vi "Build Proccess JSON creation.vi"(8 "error in (no error)":errorcluster, 9 "Project Path":path, 10 "Destination Path":path, 11 "Build Specification Name":string) -> (0 "error out":errorcluster)   [LabVIEW 2023, in "Utilities.lvlib"]
uses:
  Utilities.lvlib
  <vilib>/xml/Load XML File.vi
  <vilib>/xml/NI_XML.lvlib
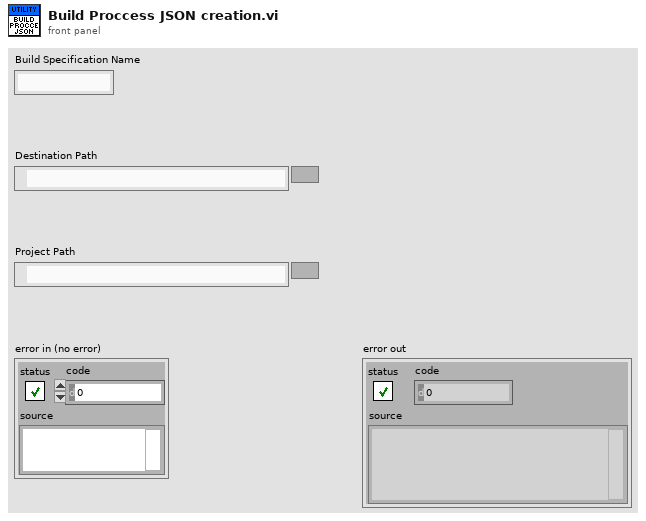
[diagram p1: front panel]
types:
  T1 = enum16{"open", "replace", "create", "open or create", "replace or create", "replace or create with confirmation"}
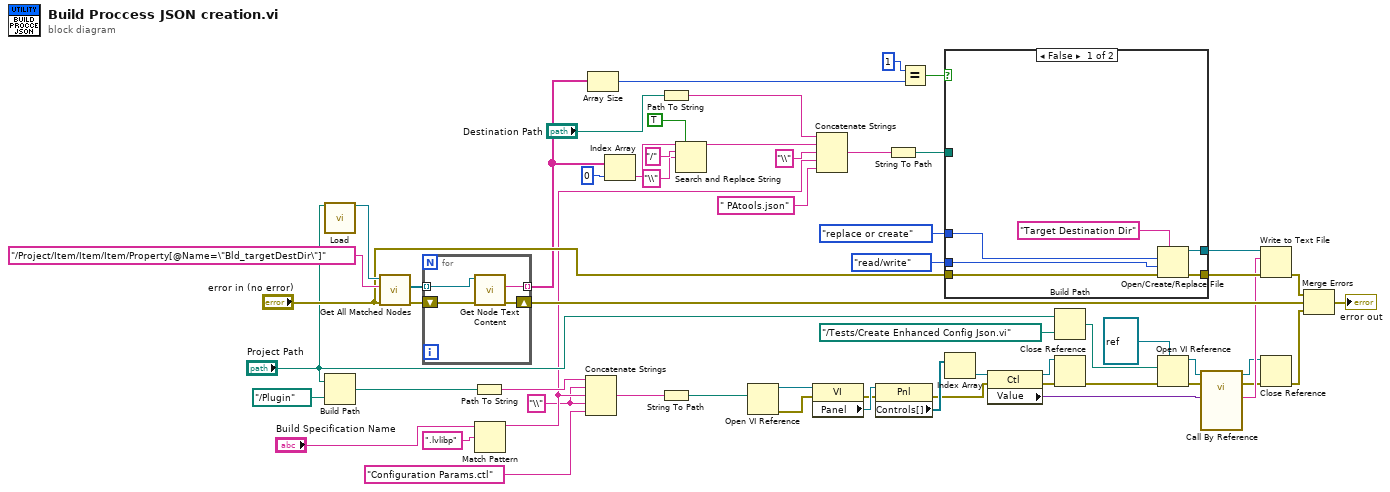
[diagram p0: block diagram]
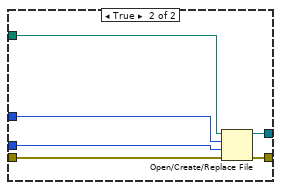
[diagram p2: hidden frame]
diagram:
  w5 = "\\" ("string")
  n1 = call-poly <vilib>:"Load.vi"("path to XML document"="Project Path") -> ("DOM document out"=w53:refnum<k20>)  [unwired: 12 in, 2 out]
  n2 = Build Path(base path="Project Path", name or relative path=path "../Plugin") -> (appended path=w1:path)
  n3 = call <vilib>:"Get All Matched Nodes.vi"("error in (no error)"="error in (no error)", "XPath expression"="/Project/Item/Item/Item/Property[@Name=\"Bld_targetDestDir\"]", "node in"=w53) -> ("error out"=w52:errorcluster, "node result array"=w47:refnum<k20>[])  [unwired: 6 in, 1 out]
  n4 = for {
    tunnel: [w63] -> w46 mode=indexing
    shift-right: [w61] -> w48
    shift-left: w52 -> [w62]
    tunnel: w47 -> [w60] mode=indexing
    n5 = call <vilib>:"Get Node Text Content.vi"("error in (no error)"=w62, "node in"=w60) -> ("error out"=w61:errorcluster, "node text"=w63:string)  [unwired: 7 in, 1 out]
  }
  n6 = Path To String(path=w1) -> (string=w7:string)
  n7 = Match Pattern(string="Build Specification Name", regular expression=".lvlibp") -> (before substring=w6:string)  [unwired: 1 in, 3 out]
  n8 = Concatenate Strings(w7, w5, w6, w5, "Configuration Params.ctl" ("string")) -> (w3:string)
  n9 = Array Size(array=w46) -> (size(s)=w44:i32)
  n10 = Index Array(array=w46, index=0) -> (element=w42:string)
  n11 = Path To String(path="Destination Path") -> (string=w58:string)
  n12 = String To Path(string=w3) -> (path=w2:path)
  n13 = Search and Replace String(replace all?=TRUE ("replace all? (F)"), input string=w42, search string="/", replace string="\\" ("replace string (\"\")")) -> (result string=w39:string)  [unwired: 4 in, 3 out]
  n14 = Open VI Reference(vi path=w2) -> (vi reference=w19:refnum<vi>, error out=w13:errorcluster)  [unwired: 5 in]
  n15 = property class="VI"(reference=w19, error in=w13) -> (error out=w12:errorcluster, "Panel"=w18:refnum<vi>)  [unwired: 1 out]
  n16 = Concatenate Strings(w58, w39, "\\" ("string"), w6, " PAtools.json" ("string")) -> (w38:string)
  n17 = property class="Pnl"(reference=w18, error in=w12) -> (error out=w11:errorcluster, "Controls[]"=w17:refnum<vi>[])  [unwired: 1 out]
  n18 = String To Path(string=w38) -> (path=w34:path)
  n19 = Equal?(x=1, y=w44) -> (x = y?=w33:bool)
  n20 = case shown="False" w33 {
    tunnel: "error in (no error)" -> [w65 w75]
    tunnel: [w66 w74] -> w37
    tunnel: [w67 w73] -> w35
    tunnel: w34 -> [_ w72]
    tunnel: T1."replace or create" ("operation (0:open)") -> [w69 w71]
    tunnel: enum16{"read/write", "read-only", "write-only"}."read/write" ("access (0:read/write)") -> [w68 w70]
    frame False {
      n21 = Open/Create/Replace File(error in=w65, prompt="Target Destination Dir", operation (0:open)=w69, access (0:read/write)=w68) -> (refnum out=w67:refnum<file>, error out=w66:errorcluster)  [unwired: 2 in, 1 out]
    }
    frame True {
      n22 = Open/Create/Replace File(file path (use dialog)=w72, error in=w75, operation (0:open)=w71, access (0:read/write)=w70) -> (refnum out=w73:refnum<file>, error out=w74:errorcluster)  [unwired: 2 in, 1 out]
    }
  }
  n23 = Index Array(array=w17) -> (element=w16:refnum<vi>)  [unwired: 1 in]
  n24 = property class="Ctl"(reference=w16, error in=w11) -> (reference out=w10:refnum<vi>, error out=w9:errorcluster, "Value"=w14:variant)
  n25 = Build Path(base path="Project Path", name or relative path=path "../Tests/Create Enhanced Config Json.vi") -> (appended path=w27:path)
  n26 = Close Reference(reference=w10, error in (no error)=w9) -> (error out=w8:errorcluster)
  n27 = Open VI Reference(type specifier VI Refnum (for type only)=refnum<vi> refnum, vi path=w27, error in (no error)=w8) -> (vi reference=w28:refnum<vi>, error out=w24:errorcluster)  [unwired: 3 in]
  n28 = call-by-ref "?"(reference=w28, error in=w24, "Value"=w14) -> (reference out=w23:refnum<vi>, error out=w22:errorcluster, "PAtools JSON"=w25:string)  [unwired: 9 in, 1 out]
  n29 = Write to Text File(file (use dialog)=w35, text=w25, error in=w37) -> (error out=w50:errorcluster)  [unwired: 1 in, 2 out]
  n30 = Close Reference(reference=w23, error in (no error)=w22) -> (error out=w21:errorcluster)
  n31 = Merge Errors(w50, w48, w21) -> (→"error out":errorcluster)
